vi "CRYDataView Set Panel Active.vi"(8 "DataView Index":i32, 11 "Selected Panel Idx In":i32) -> ()   [LabVIEW 2013]
uses:
  CRYNew View Global.vi
  SubVI/CRYMain Sub Window Global.vi
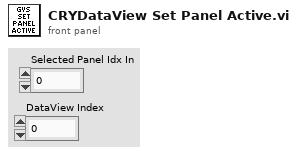
[diagram p1: front panel]
types:
  T1 = typedef "Graph Main Info Cluster.ctl" = cluster{"Selected_BarIdx":i32, "Selected_PanelIdx":i32, "Graph Main VIRef":refnum<vi>, "ToolBarClick":bool, "Spliter Ref Array":refnum<vi>[], "Panel Ref Array":refnum<vi>[], "Spliter_matrix":i32[][], "Panel_matrix":i32[][], "child_spliterIdx_matrix":i32[][], "split_pos_matrix":i32[][], "Title State":bool, "sQueueName":string, "Frame nID":i32, "Graph VIRef Array":cluster{"Graph VIRef":refnum<vi>, "Panel Idx":i32, "Frame VIRef":refnum<vi>, "Icon Ring":i32, "Graph Type":string}[], "View Type":string}
  T2 = cluster{"Graph VIRef":refnum<vi>, "Panel Idx":i32, "Frame VIRef":refnum<vi>, "Icon Ring":i32, "Graph Type":string}[]
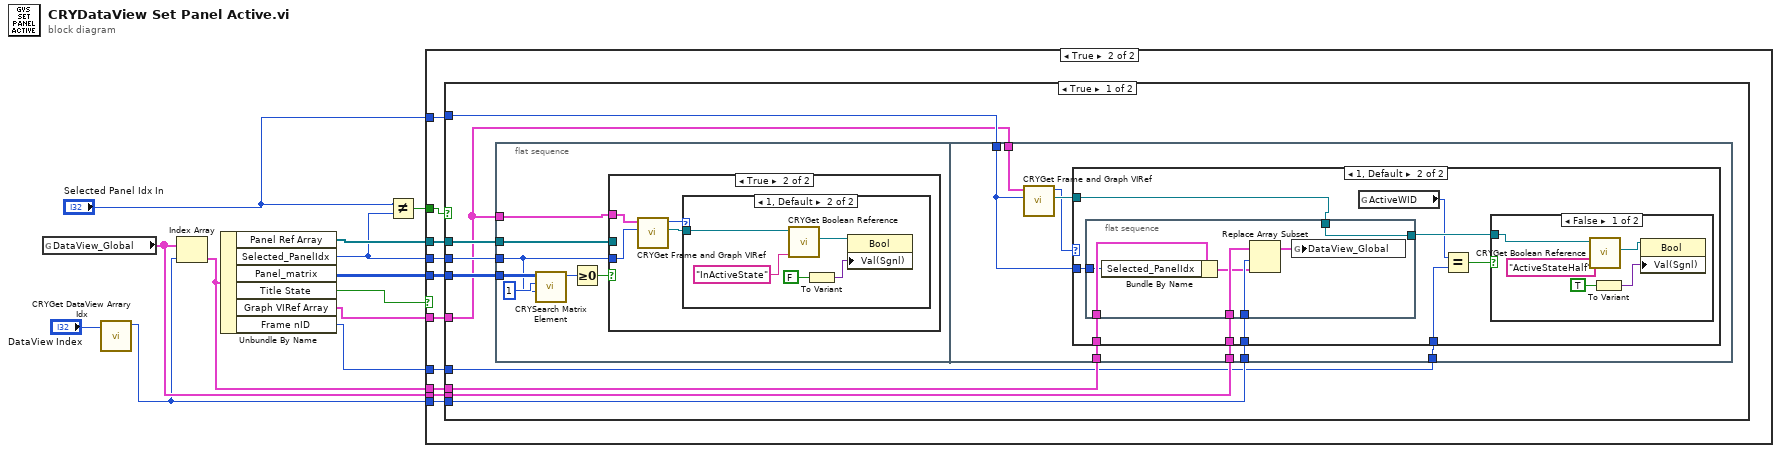
[diagram p0: block diagram]
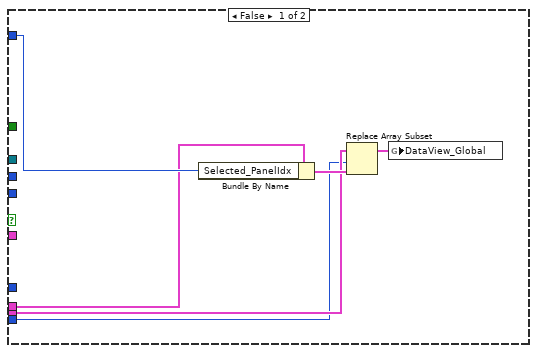
[diagram p2: hidden frame]
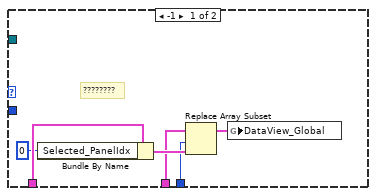
[diagram p5: hidden frame]
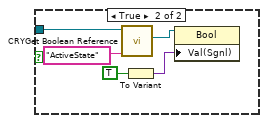
[diagram p6: hidden frame]
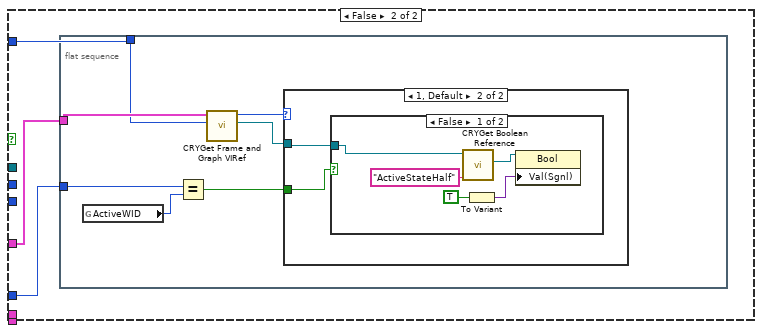
[diagram p7: hidden frame]
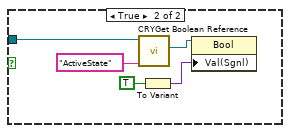
[diagram p9: hidden frame]
diagram:
  n1 = global read "CRYNew View Global.vi" "DataView_Global"() -> (w11:T1[])
  n2 = call "CRYGet DataView Arrary Idx.vi"("DataView Idx In"="DataView Index") -> ("DataView Arrary Idx out"=w7:i32)  [unwired: 10 in]
  n3 = Index Array(array=w11, index=w7) -> (element=w10:T1)
  n4 = Unbundle By Name(w10) -> ("Panel Ref Array"=w9:refnum<vi>[], "Selected_PanelIdx"=w5:i32, "Panel_matrix"=w12:i32[][], "Title State"=w3:bool, "Graph VIRef Array"=w2:T2, "Frame nID"=w1:i32)
  n5 = Not Equal?(x="Selected Panel Idx In", y=w5) -> (x != y?=w4:bool)
  n6 = case shown="True" w3 {
    tunnel: w12 -> [_ w28]
    tunnel: w11 -> [w14 w27]
    tunnel: w10 -> [w15 w26]
    tunnel: w9 -> [_ w25]
    tunnel: w7 -> [w13 w24]
    tunnel: "Selected Panel Idx In" -> [w16 w23]
    tunnel: w5 -> [_ w22]
    tunnel: w4 -> [_ w21]
    tunnel: w2 -> [_ w20]
    tunnel: w1 -> [_ w19]
    frame False {
      n7 = Bundle By Name(cluster=w15, "Selected_PanelIdx"=w16) -> (w18:T1)
      n8 = Replace Array Subset(array=w14, new element=w18, index=w13) -> (w17:T1[])
      n9 = global write "CRYNew View Global.vi" "DataView_Global"(w17) -> ()
    }
    frame True {
      n10 = case shown="True" w21 {
        tunnel: w28 -> [w37 _]
        tunnel: w27 -> [w36 _]
        tunnel: w26 -> [w35 _]
        tunnel: w25 -> [w31 _]
        tunnel: w24 -> [w34 _]
        tunnel: w23 -> [w33 w96]
        tunnel: w22 -> [w32 _]
        tunnel: w20 -> [w30 w95]
        tunnel: w19 -> [w29 w94]
        frame True {
          n11 = flat-sequence {
            tunnel: w37 -> [w44]
            tunnel: w31 -> [w40]
            tunnel: w32 -> [w39]
            tunnel: w30 -> [w38]
            tunnel: w33 -> [w57]
            tunnel: w36 -> [w61]
            tunnel: w35 -> [w60]
            tunnel: w34 -> [w59]
            tunnel: w30 -> [w58]
            tunnel: w29 -> [w54]
            frame #0 {
              n12 = call "CRYSearch Matrix Element.vi"("element"=w39, "index (row)"=1, "matrix in"=w44) -> ("index of element"=w42:i32)  [unwired: 8 in]
              n13 = Greater Or Equal To 0?(x=w42) -> (x >= 0?=w41:bool)
              n14 = case shown="True" w41 {
                tunnel: w40 -> [_ _]
                tunnel: w39 -> [_ w47]
                tunnel: w38 -> [_ w48]
                frame False {
                }
                frame True {
                  n15 = call "CRYGet Frame and Graph VIRef.vi"("Panel Idx"=w47, "Graph VIRef Array"=w48) -> ("Frame VIRef"=w46:refnum<vi>, "Graph VIRef Array Index"=w45:i32)  [unwired: 5 in, 3 out]
                  n16 = case shown="1, Default" w45 {
                    tunnel: w46 -> [_ w49]
                    frame -1 {
                    }
                    frame 1, Default {
                      n17 = call "CRYGet Boolean Reference.vi"("Label Name"="InActiveState", "VI Refnum"=w49) -> ("Boolean Ref"=w51:refnum<vi>)  [unwired: 7 in, 2 out]
                      n18 = To Variant(anything=FALSE) -> (Variant=w52:variant)
                      n19 = property class="Bool"(reference=w51, "Val(Sgnl)"=w52) -> ()  [unwired: 1 in, 2 out]
                    }
                  }
                }
              }
            }
            frame #1 {
              n20 = call "CRYGet Frame and Graph VIRef.vi"("Panel Idx"=w57, "Graph VIRef Array"=w58) -> ("Frame VIRef"=w56:refnum<vi>, "Graph VIRef Array Index"=w55:i32)  [unwired: 5 in, 3 out]
              n21 = case shown="1, Default" w55 {
                tunnel: w61 -> [w65 w76]
                tunnel: w60 -> [w63 w75]
                tunnel: w59 -> [w64 w74]
                tunnel: w57 -> [_ w73]
                tunnel: w56 -> [_ w72]
                tunnel: w54 -> [_ w68]
                frame -1 {
                  # "????????"
                  n22 = Bundle By Name(cluster=w63, "Selected_PanelIdx"=0) -> (w67:T1)
                  n23 = Replace Array Subset(array=w65, new element=w67, index=w64) -> (w66:T1[])
                  n24 = global write "CRYNew View Global.vi" "DataView_Global"(w66) -> ()
                }
                frame 1, Default {
                  n25 = flat-sequence {
                    tunnel: w76 -> [w93]
                    tunnel: w75 -> [w92]
                    tunnel: w74 -> [w91]
                    tunnel: w73 -> [w90]
                    tunnel: w72 -> [w87]
                    tunnel: [w87] -> w71
                    frame #0 {
                      n26 = Bundle By Name(cluster=w92, "Selected_PanelIdx"=w90) -> (w89:T1)
                      n27 = Replace Array Subset(array=w93, new element=w89, index=w91) -> (w88:T1[])
                      n28 = global write "CRYNew View Global.vi" "DataView_Global"(w88) -> ()
                    }
                  }
                  n29 = global read "CRYMain Sub Window Global.vi" "ActiveWID"() -> (w69:i32)
                  n30 = Equal?(x=w69, y=w68) -> (x = y?=w70:bool)
                  n31 = case shown="False" w70 {
                    tunnel: w71 -> [w77 w82]
                    frame False {
                      n32 = call "CRYGet Boolean Reference.vi"("Label Name"="ActiveStateHalf", "VI Refnum"=w77) -> ("Boolean Ref"=w80:refnum<vi>)  [unwired: 7 in, 2 out]
                      n33 = To Variant(anything=TRUE) -> (Variant=w79:variant)
                      n34 = property class="Bool"(reference=w80, "Val(Sgnl)"=w79) -> ()  [unwired: 1 in, 2 out]
                    }
                    frame True {
                      n35 = call "CRYGet Boolean Reference.vi"("Label Name"="ActiveState", "VI Refnum"=w82) -> ("Boolean Ref"=w85:refnum<vi>)  [unwired: 7 in, 2 out]
                      n36 = To Variant(anything=TRUE) -> (Variant=w84:variant)
                      n37 = property class="Bool"(reference=w85, "Val(Sgnl)"=w84) -> ()  [unwired: 1 in, 2 out]
                    }
                  }
                }
              }
            }
          }
        }
        frame False {
          n38 = flat-sequence {
            tunnel: w96 -> [w102]
            tunnel: w95 -> [w103]
            tunnel: w94 -> [w99]
            frame #0 {
              n39 = global read "CRYMain Sub Window Global.vi" "ActiveWID"() -> (w98:i32)
              n40 = Equal?(x=w99, y=w98) -> (x = y?=w97:bool)
              n41 = call "CRYGet Frame and Graph VIRef.vi"("Panel Idx"=w102, "Graph VIRef Array"=w103) -> ("Frame VIRef"=w101:refnum<vi>, "Graph VIRef Array Index"=w100:i32)  [unwired: 5 in, 3 out]
              n42 = case shown="1, Default" w100 {
                tunnel: w101 -> [_ w105]
                tunnel: w97 -> [_ w104]
                frame -1 {
                }
                frame 1, Default {
                  n43 = case shown="False" w104 {
                    tunnel: w105 -> [w106 w115]
                    frame False {
                      n44 = call "CRYGet Boolean Reference.vi"("Label Name"="ActiveStateHalf", "VI Refnum"=w106) -> ("Boolean Ref"=w109:refnum<vi>)  [unwired: 7 in, 2 out]
                      n45 = To Variant(anything=TRUE) -> (Variant=w108:variant)
                      n46 = property class="Bool"(reference=w109, "Val(Sgnl)"=w108) -> ()  [unwired: 1 in, 2 out]
                    }
                    frame True {
                      n47 = call "CRYGet Boolean Reference.vi"("Label Name"="ActiveState", "VI Refnum"=w115) -> ("Boolean Ref"=w113:refnum<vi>)  [unwired: 7 in, 2 out]
                      n48 = To Variant(anything=TRUE) -> (Variant=w112:variant)
                      n49 = property class="Bool"(reference=w113, "Val(Sgnl)"=w112) -> ()  [unwired: 1 in, 2 out]
                    }
                  }
                }
              }
            }
          }
        }
      }
    }
  }
